vi "host_logging_old.vi"() -> ()   [LabVIEW 2011]
uses:
  <vilib>/Platform/TimedLoop/XDataNode/XDataNode.xnode
  <vilib>/Platform/TimedLoop/XDataNode/nitl_modes.ctl
  <vilib>/Platform/TimedLoop/XDataNode/XDNodeRunTimeDep.lvlib
  <vilib>/Platform/TimedLoop/XDataNode/wakeup.ctl
  <vilib>/Platform/TimedLoop/XDataNode/timing_clust.ctl
  <vilib>/addons/database/NI_Database_API.lvlib
  <vilib>/Utility/error.llb/DialogType.ctl
  <vilib>/addons/database/Connection.llb/Conn ObjectReference.ctl
  Input - Cluster b2g2.ctl
  Output - Cluster b2g2.ctl
panel:
  out "source out":string
  out "code out":i32 format="%0.0f"
  out "error?":bool
  in  "db Interval [s]":u32=10 min=1 step=1
  in  "Pfad 2":path=path "C:/Git/B2G/B2G_db_rz.dsn"
  in  "DB Log":bool
  in  "stop":bool
  in  "Pfad":path=path "T:/Projekt_B2G_FABES/B2G/Messprotokolle_B2G1"
  in  "file Interval [s]":u32=60 min=1 step=1
  in  "Output - Cluster":T1 {"TS-5 [°C]" format="%#.2g"; "pHS-1 [pH]" format="%.2g"; "TS-4 [°C]" format="%#.2g"; "FS-2 [l]" format="%.2g"; "FS-1 [l]" format="%.2g"; "DS-1 [bar]" format="%#.2g"; "DFS-1 [l/min]" format="%#.2g"; "FS-3 [l]" format="%.2g"; "DFS-1 [dl]" format="%.0g"}
  in  "File Log":bool
  in  "Input - Cluster":T2 {"Dosiergeschw. [l/min]" format="%.2g"; "Füllstand  P" max=100 step=1 format="%#_3g"; "P-4 Drehzahl [%]" max=100 step=1 format="%#_3g"}
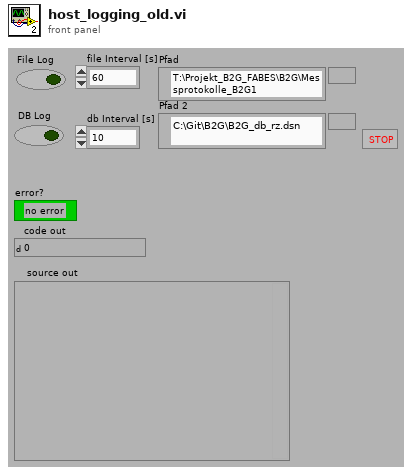
[diagram p1: front panel]
types:
  T1 = typedef "Output - Cluster b2g2.ctl" = cluster{"DFS-1 [dl]":u64, "FS-3 [l]":dbl, "DFS-1 [l/min]":dbl, "DS-1 [bar]":dbl, "V-10 ZU":bool, "V-14 ZU":bool, "FS-1 [l]":dbl, "FS-2 [l]":dbl, "TS-4 [°C]":dbl, "HS-1":bool, "V-13 [%]":u8, "V-15 [%]":u8, "P-4 [%]":u8, "Dosierung":bool, "MR Max Füllstand":bool, "MR Min Füllstand":bool, "Dosiermenge [l]":sgl, "V-14 AUF":bool, "V-10 AUF":bool, "T-1 Max Füllstand":bool, "T-1 Min Füllstand":bool, "T-2 Max Füllstand":bool, "T-2 Min Füllstand":bool, "pHS-1 [pH]":dbl, "P-4 RUN":bool, "V-33 AUF":bool, "V-33 ZU":bool, "V-34 AUF":bool, "V-34 ZU":bool, "P-4 ERR":bool, "TS-5 [°C]":dbl, "V-35 AUF":bool, "V-35 ZU":bool}
  T2 = typedef "Input - Cluster b2g2.ctl" = cluster{"V-13 [%]":u8, "V-15 [%]":u8, "Log-Target":bool, "P-4":bool, "P-4 Drehzahl [%]":u8, "Temperaturregelung":bool, "Überdruckregelung":bool, "Füllstandsregulierung":bool, "V-10":bool, "Log-Host":bool, "V-14":bool, "HS-1":bool, "Füllstand  P":sgl, "Füllstand I":sgl, "Füllstand D":sgl, "Füllstand Soll [l]":sgl, "Druck  P":sgl, "Druck I":sgl, "Druck D":sgl, "Druck Soll [bar]":sgl, "Temp Soll [°C]":sgl, "Dosierung":bool, "Dosiermenge [l]":sgl, "Dosiergeschw. [l/min]":sgl, "Tank":bool, "Hysterese [°C]":sgl, "MR Füllstandsüberwachung":bool, "Tank Füllstandsüberwachung":bool, "Log Target [ms]":u32, "Log Host [s]":u32, "Zirkulation EIN [min]":u8, "Zirkulation AUS [min]":u8, "Zirkulation":bool, "V-33":bool, "V-34":bool, "V-35":bool}
  T3 = typedef "NI_Database_API.lvlib/Conn ObjectReference.ctl" = refnum<k1>
  T4 = cluster{"file reference":refnum<file>, "file timing":i64, "db timing":i64, "DFS-1":u64, "db reference":T3, "P4":bool, "P5":bool, "file":bool, "db":bool, "data refnum":refnum<k21>, "input refnum":refnum<k21>, "feeding":bool, "feeding start volume":u64, "feeding start time":timestamp, "flashing":bool, "flashing start volume":u64, "flashing start time":timestamp, "V-33":bool, "V-34":bool, "V-15":u8, "V-13":u8}
  T5 = typedef "XDNodeRunTimeDep.lvlib/timing_clust.ctl" = cluster{"Expected End [f-1]":u64, "Actual End [f-1]":u64, "Finished Late? [f-1]":bool, "Expected End [i-1]":u64, "Actual End [i-1]":u64, "Finished Late? [i-1]":bool, "Expected Start [i]":u64, "Actual Start [i]":u64, "Expected Start [f]":u64, "Actual Start [f]":u64, "Source Name":string, "Structure Name":string, "Period":i64, "Deadline":i64, "Offset":i64, "Start":i64, "Priority":i32, "Timeout":i32, "Mode":T6, "Wakeup Reason":T7, "Error":errorcluster, "Source Type":string, "Secondary Source Type":string, "Global End Time":u64, "Global Start Time":u64, "Frame Duration":u64, "Iteration Duration":u64, "Assigned CPU":i32, "I/O Scan Engine Mode":u32}
  T6 = typedef "XDNodeRunTimeDep.lvlib/nitl_modes.ctl" = enum32{"No Change", "Process missed periods, maintain original phase", "Discard missed periods, maintain original phase", "Process missed periods, ignore original phase", "Discard missed periods, ignore original phase"}
  T7 = typedef "XDNodeRunTimeDep.lvlib/wakeup.ctl" = enum32{"Normal", "Aborted", "Asynchronous wakeup", "Timing source error", "Timed loop error", "Timeout"}
  T8 = typedef "DialogType.ctl" = u16
  T9 = cluster{"seconds since 1Jan1904":timestamp, "code":i32, "source":string}
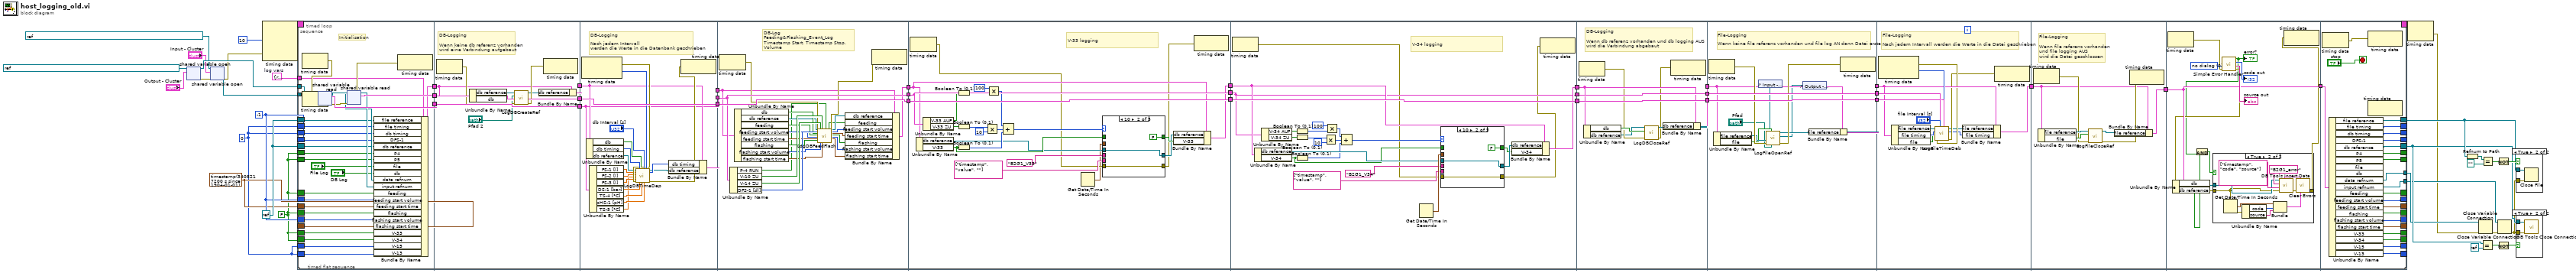
[diagram p0: block diagram]
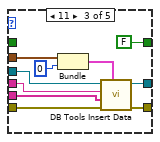
[diagram p5: hidden frame]
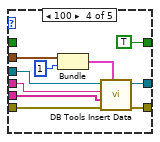
[diagram p6: hidden frame]
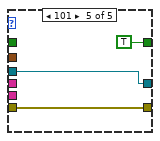
[diagram p7: hidden frame]
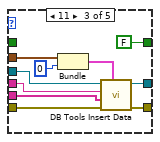
[diagram p9: hidden frame]
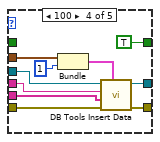
[diagram p10: hidden frame]
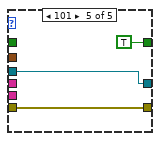
[diagram p11: hidden frame]
diagram:
  w20 = T4 {"file reference"=refnum, "file timing"=0, "db timing"=0, "DFS-1"=0, "db reference"=refnum, "P4"=FALSE, "P5"=FALSE, "file"=FALSE, "db"=FALSE, "data refnum"="ni.var.psp://10.27.40.21/variables - network - RT (separate)/data - network", "input refnum"="ni.var.psp://10.27.40.21/variables - network - RT (separate)/data - network", "feeding"=FALSE, "feeding start volume"=0, "feeding start time"=timestamp(0 s since 1904-01-01), "flashing"=FALSE, "flashing start volume"=0, "flashing start time"=timestamp(0 s since 1904-01-01), "V-33"=FALSE, "V-34"=FALSE, "V-15"=0, "V-13"=0}  # log vars
  w3 = timestamp(3408217200 s since 1904-01-01) ("Time Stamp")
  w1 = FALSE ("P5")
  w4 = -1
  w2 = i64 0 ("Actual Start [i]")
  w18 = refnum<k0> refnum
  n1 = shared-variable-open(refnum<k21> "ni.var.psp://10.27.40.21/variables - network - RT (separate)/data - network" ("shared variable refnum in"), "Output - Cluster") -> (w17:refnum<k21>, w11:errorcluster)  [unwired: 2 in]
  n2 = shared-variable-open(refnum<k21> "ni.var.psp://10.27.40.21/variables - network - RT (separate)/input - network" ("shared variable refnum in"), w11, "Input - Cluster") -> (w12:refnum<k21>, w10:errorcluster)  [unwired: 1 in]
  n3 = node-c288(i64 10 ("Period"), w10) -> (w31:T5)  [unwired: 2 in]
  n4 = timed-loop {
    timing: w31 -> [_]
    timing-out: [_] -> w30
    shift-right: [w69] -> w26
    shift-left: w18 -> [w70]
    shift-right: [w67] -> _
    shift-left: w2 -> [w68]
    shift-right: [w65] -> _
    shift-left: w2 -> [w66]
    tunnel: w20 -> [w64]
    shift-right: [w63] -> _
    shift-left: w4 -> [w52]
    shift-right: [w62] -> w21
    shift-left: w18 -> [w61]
    shift-right: [w60] -> _
    shift-left: w1 -> [w59]
    shift-right: [w58] -> _
    shift-left: w1 -> [w57]
    tunnel: w17 -> [w56]
    tunnel: w12 -> [w55]
    tunnel: [w54] -> w9
    tunnel: [w53] -> w8
    shift-right: [w51] -> _
    shift-left: w1 -> [w50]
    shift-right: [w49] -> _
    shift-left: w1 -> [w48]
    shift-right: [w47] -> _
    shift-left: w4 -> [w46]
    shift-right: [w45] -> _
    shift-left: w4 -> [w44]
    shift-right: [w43] -> _
    shift-left: w3 -> [w42]
    shift-right: [w41] -> _
    shift-left: w3 -> [w40]
    shift-right: [w39] -> _
    shift-left: w2 -> [w33]
    shift-right: [w38] -> _
    shift-left: w2 -> [w32]
    shift-right: [w37] -> _
    shift-left: w1 -> [w34]
    shift-right: [w36] -> _
    shift-left: w1 -> [w35]
    stop <- "stop" stop-if-true
    n5 = timed-sequence {
      timing: _ -> [_]
      timing-out: _ -> [_]
      tunnel: w70 -> [w136]
      tunnel: [w135] -> w69
      tunnel: w68 -> [w134]
      tunnel: [w133] -> w67
      tunnel: w66 -> [w132]
      tunnel: [w131] -> w65
      tunnel: w64 -> [w130]
      tunnel: [w129] -> w63
      tunnel: [w128] -> w62
      tunnel: w61 -> [w127]
      tunnel: [w126] -> w60
      tunnel: w59 -> [w125]
      tunnel: [w124] -> w58
      tunnel: w57 -> [w123]
      tunnel: w56 -> [w116]
      tunnel: w55 -> [w115]
      tunnel: [w114] -> w54
      tunnel: [w113] -> w53
      tunnel: w52 -> [w105]
      tunnel: [w101] -> w51
      tunnel: w50 -> [w100]
      tunnel: [w99] -> w49
      tunnel: w48 -> [w98]
      tunnel: [w97] -> w47
      tunnel: w46 -> [w96]
      tunnel: [w95] -> w45
      tunnel: w44 -> [w94]
      tunnel: [w93] -> w43
      tunnel: w42 -> [w92]
      tunnel: [w91] -> w41
      tunnel: w40 -> [w90]
      tunnel: [w84] -> w39
      tunnel: [w83] -> w38
      tunnel: [w82] -> w37
      tunnel: [w81] -> w36
      tunnel: w35 -> [w80]
      tunnel: w34 -> [w79]
      tunnel: w33 -> [w78]
      tunnel: w32 -> [w77]
      n6 = timed-flat-sequence {
        tunnel: w134 -> [w141]
        tunnel: w136 -> [w139]
        tunnel: [w163] -> w122
        tunnel: [w162] -> w120
        tunnel: w132 -> [w140]
        tunnel: w130 -> [w138]
        tunnel: [w137] -> w118
        tunnel: w127 -> [w143]
        tunnel: w125 -> [w144]
        tunnel: w123 -> [w145]
        tunnel: w116 -> [w166]
        tunnel: w115 -> [w164]
        tunnel: w105 -> [w142]
        tunnel: w100 -> [w150]
        tunnel: w98 -> [w153]
        tunnel: w96 -> [w151]
        tunnel: w94 -> [w154]
        tunnel: w92 -> [w155]
        tunnel: w90 -> [w152]
        tunnel: w80 -> [w156]
        tunnel: w79 -> [w157]
        tunnel: w78 -> [w158]
        tunnel: w77 -> [w159]
        tunnel: w122 -> [w181]
        tunnel: [w181] -> w121
        tunnel: w120 -> [w180]
        tunnel: [w180] -> w119
        tunnel: w118 -> [w176]
        tunnel: [w175] -> w117
        tunnel: w121 -> [w194]
        tunnel: [w194] -> w104
        tunnel: w119 -> [w206]
        tunnel: [w206] -> w103
        tunnel: w117 -> [w195]
        tunnel: [w203] -> w102
        tunnel: w104 -> [w236]
        tunnel: [w236] -> w87
        tunnel: w103 -> [w237]
        tunnel: [w237] -> w86
        tunnel: w102 -> [w224]
        tunnel: [w230] -> w85
        tunnel: w87 -> [w264]
        tunnel: [w264] -> w76
        tunnel: w86 -> [w265]
        tunnel: [w265] -> w74
        tunnel: w85 -> [w263]
        tunnel: [w262] -> w72
        tunnel: w76 -> [w302]
        tunnel: [w302] -> w75
        tunnel: w74 -> [w322]
        tunnel: [w322] -> w73
        tunnel: w72 -> [w303]
        tunnel: [w304] -> w71
        tunnel: w75 -> [w365]
        tunnel: [w365] -> w112
        tunnel: w73 -> [w364]
        tunnel: [w364] -> w110
        tunnel: w71 -> [w362]
        tunnel: [w361] -> w108
        tunnel: w112 -> [w382]
        tunnel: [w382] -> w111
        tunnel: w110 -> [w381]
        tunnel: [w381] -> w109
        tunnel: w108 -> [w376]
        tunnel: [w375] -> w107
        tunnel: w111 -> [w399]
        tunnel: w109 -> [w398]
        tunnel: w107 -> [w395]
        tunnel: [w396] -> w106
        tunnel: w106 -> [w409]
        tunnel: [w408] -> w89
        tunnel: w89 -> [w425]
        tunnel: [w425] -> w88
        tunnel: [w463] -> w131
        tunnel: [w462] -> w133
        tunnel: [w464] -> w135
        tunnel: w88 -> [w465]
        tunnel: [w461] -> w129
        tunnel: [w460] -> w128
        tunnel: [w459] -> w126
        tunnel: [w458] -> w124
        tunnel: [w457] -> w114
        tunnel: [w456] -> w113
        tunnel: [w455] -> w101
        tunnel: [w452] -> w99
        tunnel: [w454] -> w97
        tunnel: [w451] -> w95
        tunnel: [w450] -> w93
        tunnel: [w453] -> w91
        tunnel: [w447] -> w84
        tunnel: [w446] -> w83
        tunnel: [w448] -> w82
        tunnel: [w449] -> w81
        frame #0 {
          # "Initialisation"
          n7 = node-c288() -> (w165:errorcluster)  [unwired: 1 in]
          n8 = shared-variable-read(w166, w165) -> (w148:refnum<k21>, w161:errorcluster, w163:T1)  [unwired: 1 out]
          n9 = shared-variable-read(w164, w161) -> (w149:refnum<k21>, w160:errorcluster, w162:T2)  [unwired: 1 out]
          n10 = Bundle By Name(cluster=w138, "file reference"=w139, "file timing"=w140, "db timing"=w141, "DFS-1"=w142, "db reference"=w143, "P4"=w144, "P5"=w145, "file"="File Log", "db"="DB Log", "data refnum"=w148, "input refnum"=w149, "feeding"=w150, "feeding start volume"=w151, "feeding start time"=w152, "flashing"=w153, "flashing start volume"=w154, "flashing start time"=w155, "V-33"=w156, "V-34"=w157, "V-15"=w158, "V-13"=w159) -> (w137:T4)
          n11 = node-c288(w160) -> ()  [unwired: 1 out]
        }
        frame #1 {
          # "DB-Logging\n\nWenn keine db referenz vorhanden\nwird eine Verbindung aufgebaut"
          n12 = node-c288() -> (w178:errorcluster)  [unwired: 1 in]
          n13 = Unbundle By Name(w176) -> ("db reference"=w179:T3, "db"=w173:bool)
          n14 = call "LogDBCreateRef.vi"("error in (no error)"=w178, "db"=w173, "Pfad in"="Pfad 2", "Refnum in"=w179) -> ("error out"=w177:errorcluster, "Refnum out"=w174:T3)  [unwired: 6 in]
          n15 = Bundle By Name(cluster=w176, "db reference"=w174) -> (w175:T4)
          n16 = node-c288(w177) -> ()  [unwired: 1 out]
        }
        frame #2 {
          # "DB-Logging\n\nNach jedem Intervall \nwerden die Werte in die Datenbank geschrieben"
          n17 = node-c288() -> (w200:errorcluster, w204:i64)  [unwired: 1 in]
          n18 = Unbundle By Name(w195) -> ("db"=w196:bool, "db timing"=w202:i64, "db reference"=w197:T3)
          n19 = Unbundle By Name(w194) -> ("FS-1 [l]"=w193:dbl, "FS-2 [l]"=w192:dbl, "FS-3 [l]"=w191:dbl, "DS-1 [bar]"=w190:dbl, "TS-4 [°C]"=w189:dbl, "pHS-1 [pH]"=w188:dbl, "TS-5 [°C]"=w187:dbl)
          n20 = call "LogDBTimeDep.vi"("Refnum in"=w197, "FS-1 [l]"=w193, "FS-2 [l]"=w192, "TS-5 [°C]"=w187, "FS-3 [l]"=w191, "error in (no error)"=w200, "db timing"=w202, "DS-1 [bar]"=w190, "db"=w196, "TS-4 [°C]"=w189, "db Interval [s]"="db Interval [s]", "pHS-1 [pH]"=w188, "Actual Start [f] in"=w204) -> ("Refnum out"=w198:T3, "Actual Start [f] out"=w201:i64, "error out"=w199:errorcluster)  [unwired: 4 in]
          n21 = Bundle By Name(cluster=w195, "db timing"=w201, "db reference"=w198) -> (w203:T4)
          n22 = node-c288(w199) -> ()  [unwired: 1 out]
        }
        frame #3 {
          # "DB-Log\nFeeding&Flashing_Event_Log\nTimestamp Start, Timestamp Stop, Volume"
          n23 = node-c288() -> (w232:errorcluster)  [unwired: 1 in]
          n24 = Unbundle By Name(w236) -> ("P-4 RUN"=w213:bool, "V-10 ZU"=w234:bool, "V-14 ZU"=w233:bool, "DFS-1 [dl]"=w235:u64)
          n25 = Unbundle By Name(w224) -> ("db"=w227:bool, "db reference"=w226:T3, "feeding"=w214:bool, "feeding start volume"=w225:u64, "feeding start time"=w223:timestamp, "flashing"=w215:bool, "flashing start volume"=w217:u64, "flashing start time"=w216:timestamp)
          n26 = call "LogDBFeedFlash.vi"("Refnum in"=w226, "value volume [dl]"=w235, "enable"=w227, "feeding"=w214, "feeding start volume"=w225, "feeding start time"=w223, "flashing"=w215, "error in"=w232, "valve t-2 close"=w233, "flashing start volume"=w217, "valve t-1 close"=w234, "flashing start time"=w216, "Pump"=w213) -> ("feeding"=w228:bool, "Refnum out"=w229:T3, "feeding start volume"=w221:u64, "feeding start time"=w222:timestamp, "flashing"=w219:bool, "flashing start volume"=w218:u64, "flashing start time"=w220:timestamp, "error out"=w231:errorcluster)  [unwired: 7 in]
          n27 = Bundle By Name(cluster=w224, "db reference"=w229, "feeding"=w228, "feeding start volume"=w221, "feeding start time"=w222, "flashing"=w219, "flashing start volume"=w218, "flashing start time"=w220) -> (w230:T4)
          n28 = node-c288(w231) -> ()  [unwired: 1 out]
        }
        frame #4 {
          # "V-33 logging"
          n29 = node-c288() -> (w245:errorcluster)  [unwired: 1 in]
          n30 = Unbundle By Name(w263) -> ("db reference"=w250:T3, "V-33"=w252:bool)
          n31 = Unbundle By Name(w264) -> ("V-33 AUF"=w249:bool, "V-33 ZU"=w248:bool)
          n32 = Boolean To (0,1)(Boolean=w249) -> (0, 1=w261:i16)
          n33 = Boolean To (0,1)(Boolean=w248) -> (0, 1=w257:i16)
          n34 = Boolean To (0,1)(Boolean=w252) -> (0, 1=w258:i16)
          n35 = Multiply(x=w257, y=i16 10 ("x")) -> (x*y=w255:i16)
          n36 = Multiply(x=i16 100, y=w261) -> (x*y=w259:i16)
          n37 = Compound Arithmetic op=ADD(w259, w255, w258) -> (w254:i16)
          n38 = Get Date/Time In Seconds() -> (seconds since 1Jan1904=w243:timestamp)
          n39 = case shown="10" w254 {
            tunnel: [w268 FALSE ("V-33") FALSE ("V-33") TRUE ("V-33") TRUE ("V-33")] -> w253
            tunnel: w252 -> [w268 _ _ _ _]
            tunnel: [w267 w270 w277 w287 w293] -> w251
            tunnel: w250 -> [w267 w270 w278 w288 w293]
            tunnel: "B2G1_V33" ("table") -> [_ _ w280 w290 _]
            tunnel: string[] ["timestamp", "value", ""] ("columns") -> [_ _ w279 w289 _]
            tunnel: w245 -> [w266 w269 w276 w286 w292]
            tunnel: [w266 w269 w275 w285 w292] -> w244
            tunnel: w243 -> [_ _ w274 w284 _]
            frame 0, Default {
            }
            frame 10 {
            }
            frame 11 {
              n40 = Bundle("seconds since 1Jan1904"=w274, 0) -> (w273:cluster{"seconds since 1Jan1904":timestamp, i32})  [unwired: 1 in]
              n41 = call <vilib>:"DB Tools Insert Data.vi"("data"=w273, "error in (no error)"=w276, "columns"=w279, "table"=w280, "connection reference"=w278) -> ("error out"=w275:errorcluster, "connection reference out"=w277:T3)  [unwired: 5 in]
            }
            frame 100 {
              n42 = Bundle("seconds since 1Jan1904"=w284, 1) -> (w283:cluster{"seconds since 1Jan1904":timestamp, i32})  [unwired: 1 in]
              n43 = call <vilib>:"DB Tools Insert Data.vi"("data"=w283, "error in (no error)"=w286, "columns"=w289, "table"=w290, "connection reference"=w288) -> ("error out"=w285:errorcluster, "connection reference out"=w287:T3)  [unwired: 5 in]
            }
            frame 101 {
            }
          }
          n44 = Bundle By Name(cluster=w263, "db reference"=w251, "V-33"=w253) -> (w262:T4)
          n45 = node-c288(w244) -> ()  [unwired: 1 out]
        }
        frame #5 {
          # "V-34 logging"
          n46 = node-c288() -> (w301:errorcluster)  [unwired: 1 in]
          n47 = Unbundle By Name(w303) -> ("db reference"=w316:T3, "V-34"=w314:bool)
          n48 = Unbundle By Name(w302) -> ("V-34 AUF"=w317:bool, "V-34 ZU"=w318:bool)
          n49 = Boolean To (0,1)(Boolean=w317) -> (0, 1=w305:i16)
          n50 = Boolean To (0,1)(Boolean=w318) -> (0, 1=w309:i16)
          n51 = Boolean To (0,1)(Boolean=w314) -> (0, 1=w308:i16)
          n52 = Multiply(x=w309, y=i16 10 ("x")) -> (x*y=w311:i16)
          n53 = Multiply(x=i16 100, y=w305) -> (x*y=w307:i16)
          n54 = Compound Arithmetic op=ADD(w307, w311, w308) -> (w312:i16)
          n55 = Get Date/Time In Seconds() -> (seconds since 1Jan1904=w321:timestamp)
          n56 = case shown="10" w312 {
            tunnel: [w325 FALSE ("V-33") FALSE ("V-33") TRUE ("V-33") TRUE ("V-33")] -> w313
            tunnel: w314 -> [w325 _ _ _ _]
            tunnel: [w324 w327 w334 w344 w350] -> w315
            tunnel: w316 -> [w324 w327 w335 w345 w350]
            tunnel: "B2G1_V34" ("table") -> [_ _ w337 w347 _]
            tunnel: string[] ["timestamp", "value", ""] ("columns") -> [_ _ w336 w346 _]
            tunnel: w301 -> [w323 w326 w333 w343 w349]
            tunnel: [w323 w326 w332 w342 w349] -> w300
            tunnel: w321 -> [_ _ w331 w341 _]
            frame 0, Default {
            }
            frame 10 {
            }
            frame 11 {
              n57 = Bundle("seconds since 1Jan1904"=w331, 0) -> (w330:cluster{"seconds since 1Jan1904":timestamp, i32})  [unwired: 1 in]
              n58 = call <vilib>:"DB Tools Insert Data.vi"("data"=w330, "error in (no error)"=w333, "columns"=w336, "table"=w337, "connection reference"=w335) -> ("error out"=w332:errorcluster, "connection reference out"=w334:T3)  [unwired: 5 in]
            }
            frame 100 {
              n59 = Bundle("seconds since 1Jan1904"=w341, 1) -> (w340:cluster{"seconds since 1Jan1904":timestamp, i32})  [unwired: 1 in]
              n60 = call <vilib>:"DB Tools Insert Data.vi"("data"=w340, "error in (no error)"=w343, "columns"=w346, "table"=w347, "connection reference"=w345) -> ("error out"=w342:errorcluster, "connection reference out"=w344:T3)  [unwired: 5 in]
            }
            frame 101 {
            }
          }
          n61 = Bundle By Name(cluster=w303, "db reference"=w315, "V-34"=w313) -> (w304:T4)
          n62 = node-c288(w300) -> ()  [unwired: 1 out]
        }
        frame #6 {
          # "DB-Logging\n\nWenn db referenz vorhanden und db logging AUS\nwird die Verbindung abgebaut"
          n63 = node-c288() -> (w359:errorcluster)  [unwired: 1 in]
          n64 = Unbundle By Name(w362) -> ("db"=w360:bool, "db reference"=w357:T3)
          n65 = call "LogDBCloseRef.vi"("error in (no error)"=w359, "enable"=w360, "Refnum in"=w357) -> ("error out"=w358:errorcluster, "Refnum out"=w363:T3)  [unwired: 7 in]
          n66 = Bundle By Name(cluster=w362, "db reference"=w363) -> (w361:T4)
          n67 = node-c288(w358) -> ()  [unwired: 1 out]
        }
        frame #7 {
          # "File-Logging\n\nWenn keine file referenz vorhanden und file log AN dann Datei erstellen"
          n68 = node-c288() -> (w380:errorcluster)  [unwired: 1 in]
          n69 = Unbundle By Name(w376) -> ("file reference"=w379:refnum<file>, "file"=w378:bool)
          n70 = control-ref of="Input - Cluster"() -> (w373:refnum<vi>)
          n71 = control-ref of="Output - Cluster"() -> (w372:refnum<vi>)
          n72 = call "LogFileOpenRef.vi"("Pfad"="Pfad", "file"=w378, "error in (no error)"=w380, "file reference"=w379, "Output - Cluster"=w372, "Cluster in"=w373) -> ("error out"=w377:errorcluster, "Byte Stream File out"=w374:refnum<file>)  [unwired: 4 in]
          n73 = Bundle By Name(cluster=w376, "file reference"=w374) -> (w375:T4)
          n74 = node-c288(w377) -> ()  [unwired: 1 out]
        }
        frame #8 {
          # "File-Logging\n\nNach jedem Intervall werden die Werte in die Datei geschrieben"
          n75 = node-c288() -> (w391:errorcluster, w397:i64)  [unwired: 1 in]
          n76 = Unbundle By Name(w395) -> ("file reference"=w392:refnum<file>, "file timing"=w394:i64, "file"=w393:bool)
          n77 = call "LogFileTimeDeb.vi"("Input - Cluster"=w398, "Actual Start [f] in"=w397, "Output - Cluster"=w399, "file Interval [s]"="file Interval [s]", "error in (no error)"=w391, "file"=w393, "file timing"=w394, "Byte Stream File in"=w392) -> ("error out"=w390:errorcluster, "Actual Start [f] out"=w388:i64, "Byte Stream File out"=w389:refnum<file>)  [unwired: 1 in]
          n78 = Bundle By Name(cluster=w395, "file reference"=w389, "file timing"=w388) -> (w396:T4)
          n79 = node-c288(w390) -> ()  [unwired: 1 out]
        }
        frame #9 {
          # "File-Logging\n\nWenn file referenz vorhanden \nund file logging AUS\nwird die Datei geschlossen"
          n80 = node-c288() -> (w411:errorcluster)  [unwired: 1 in]
          n81 = Unbundle By Name(w409) -> ("file reference"=w413:refnum<file>, "file"=w412:bool)
          n82 = call "LogFileCloseRef.vi"("error in (no error)"=w411, "file"=w412, "Byte Stream File in"=w413) -> ("error out"=w410:errorcluster, "Byte Stream File out"=w407:refnum<file>)  [unwired: 7 in]
          n83 = Bundle By Name(cluster=w409, "file reference"=w407) -> (w408:T4)
          n84 = node-c288(w410) -> ()  [unwired: 1 out]
        }
        frame #10 {
          w428 = T8 0 items=["no dialog", "OK message", "continue or stop message", "OK message + warnings", "continue/stop + warnings"] ("type of dialog (OK msg:1)")
          n85 = node-c288() -> (w426:errorcluster)  [unwired: 1 in]
          n86 = Unbundle By Name(w425) -> ("db"=w422:bool, "db reference"=w420:T3)
          n87 = call <vilib>:"Simple Error Handler.vi"("type of dialog (OK msg:1)"=w428, "error in (no error)"=w426) -> ("error?"=w419:bool, "code out"=→"code out":i32, "source out"=→"source out":string, "error out"=w424:errorcluster)  [unwired: 3 in, 1 out]
          "error?" <- w419
          n88 = And(x=w422, y=w419) -> (x .and. y?=w421:bool)
          n89 = case shown="True" w421 {
            tunnel: w424 -> [w430 w434]
            tunnel: [w430 w431] -> w423
            tunnel: w420 -> [_ w437]
            frame False {
            }
            frame True {
              n90 = Get Date/Time In Seconds() -> (seconds since 1Jan1904=w435:timestamp)
              n91 = Unbundle By Name(w434) -> ("code"=w433:i32, "source"=w432:string)
              n92 = Bundle("seconds since 1Jan1904"=w435, "code"=w433, "source"=w432) -> (w436:T9)  [unwired: 1 in]
              n93 = call <vilib>:"DB Tools Insert Data.vi"("data"=w436, "error in (no error)"=w434, "columns"=string[] ["timestamp", "code", "source"], "table"="B2G1_error", "connection reference"=w437) -> ("error out"=w438:errorcluster)  [unwired: 5 in, 1 out]
              n94 = call <vilib>:"Clear Errors.vi"("error in (no error)"=w438) -> ("error out"=w431:errorcluster)  [unwired: 6 in]
            }
          }
          n95 = node-c288(w423) -> ()  [unwired: 1 out]
        }
        frame #11 {
          n96 = node-c288() -> (w466:errorcluster)  [unwired: 1 in]
          n97 = Unbundle By Name(w465) -> ("file reference"=w464:refnum<file>, "file timing"=w463:i64, "db timing"=w462:i64, "DFS-1"=w461:u64, "db reference"=w460:T3, "P4"=w459:bool, "P5"=w458:bool, "data refnum"=w457:refnum<k21>, "input refnum"=w456:refnum<k21>, "feeding"=w455:bool, "feeding start volume"=w454:u64, "feeding start time"=w453:timestamp, "flashing"=w452:bool, "flashing start volume"=w451:u64, "flashing start time"=w450:timestamp, "V-33"=w449:bool, "V-34"=w448:bool, "V-15"=w447:u8, "V-13"=w446:u8)  [unwired: 2 out]
          n98 = node-c288(w466) -> ()  [unwired: 1 out]
        }
      }
    }
    n99 = node-c288() -> ()  [unwired: 1 in, 1 out]
    n100 = node-c288() -> ()  [unwired: 1 in, 1 out]
  }
  n101 = node-c288(w30) -> (w7:errorcluster)
  n102 = Refnum to Path(1:w26) -> (0:w19:path)
  n103 = Close Variable Connection(8:w7, 11:w9) -> (0:w6:errorcluster)
  n104 = Equal?(x=w21, y=refnum<k0> refnum) -> (x = y?=w24:bool)
  n105 = Equal?(x=w19, y=path "") -> (x = y?=w27:bool)
  n106 = Not(x=w27) -> (.not. x?=w28:bool)
  n107 = Not(x=w24) -> (.not. x?=w22:bool)
  n108 = Close Variable Connection(8:w6, 11:w8) -> (0:w5:errorcluster)
  n109 = case shown="True" w28 {
    tunnel: w26 -> [_ w476]
    tunnel: w5 -> [_ w475]
    frame False {
    }
    frame True {
      n110 = Close File(refnum=w476, error in=w475) -> ()  [unwired: 2 out]
    }
  }
  n111 = case shown="True" w22 {
    tunnel: w5 -> [_ w478]
    tunnel: w21 -> [_ w477]
    frame False {
    }
    frame True {
      n112 = call <vilib>:"DB Tools Close Connection.vi"("error in (no error)"=w478, "connection reference"=w477) -> ()  [unwired: 5 in, 1 out]
    }
  }
